vi "VCI Set User Key.vi"(8 "error in (no error)":errorcluster, 9 "pUserKey":string, 10 "DevIndex":i32, 11 "DevType":i32) -> (0 "error out":errorcluster, 3 "function return":i32)   [LabVIEW 2012, in "ControlCAN.lvlib"]
doc: "int WINAPI VCI_SetUserKey(int DevType,int DevIndex,unsigned char* pUserKey);"
uses:
  ControlCAN.lvlib
  Ginkgo_Driver.dll
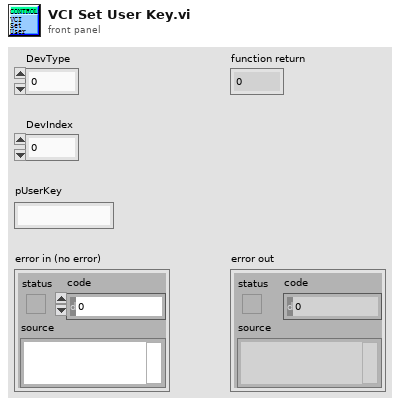
[diagram p1: front panel]
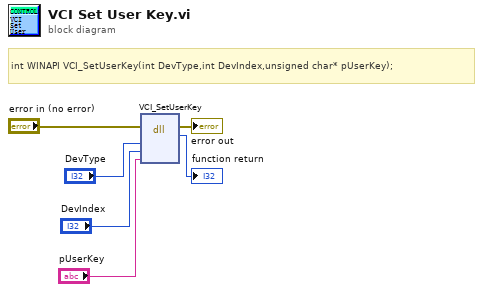
[diagram p0: block diagram]
diagram:
  # "int WINAPI VCI_SetUserKey(int DevType,int DevIndex,unsigned char* pUserKey);"
  n1 = dll-call lib="E:/Project/vt_ginkgo/truck/Ginkgo Driver/vs2010/Ginkgo_USB-I2C_API_v2.0.3.0/lib/labview_32bit/ControlCAN/Ginkgo_Driver.*" fn="VCI_SetUserKey"(error in="error in (no error)", "DevType"="DevType", "DevIndex"="DevIndex", "pUserKey"="pUserKey") -> (error out=→"error out":errorcluster, →"function return":i32)  [unwired: 5 in, 1 out]
